vi "temp.vi"() -> ()   [LabVIEW 2009]
panel:
  out "dll path":path
  out "path":path
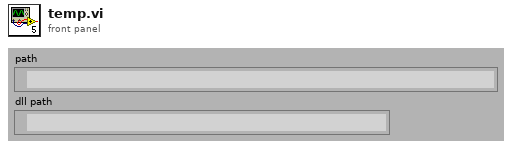
[diagram p1: front panel]
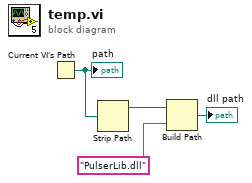
[diagram p0: block diagram]
diagram:
  n1 = Current VI's Path() -> (path=w4:path)
  "path" <- w4
  n2 = Strip Path(path=w4) -> (stripped path=w3:path)  [unwired: 1 out]
  n3 = Build Path(base path=w3, name or relative path="PulserLib.dll") -> (appended path=→"dll path":path)
